vi "VMUIAsync_Viewer.vi"(6 "SetList VariableManager ref":refnum<vi>, 10 "SubPanelRef":refnum<vi>, 11 "VariableManagerRef in":refnum<vi>) -> ()   [LabVIEW 2013]
doc: "Asynchronously call VMUI.vi with the given input. The caller process will not be blocked."
uses:
  VariableManager/VariableManager.lvclass
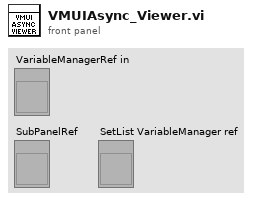
[diagram p1: front panel]
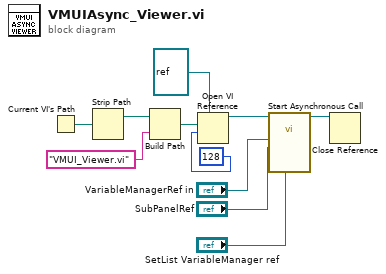
[diagram p0: block diagram]
diagram:
  n1 = Current VI's Path() -> (path=w9:path)
  n2 = Strip Path(path=w9) -> (stripped path=w10:path)  [unwired: 1 out]
  n3 = Build Path(base path=w10, name or relative path="VMUI_Viewer.vi") -> (appended path=w8:path)
  n4 = Open VI Reference(type specifier VI Refnum (for type only)=refnum<vi> refnum, vi path=w8, options=128) -> (vi reference=w4:refnum<vi>)  [unwired: 3 in, 1 out]
  n5 = call-by-ref "Start Asynchronous Call"(reference=w4, "SetList VariableManager Ref in"="SetList VariableManager ref", "SubPanelRef"="SubPanelRef", "VariableManagerRef in"="VariableManagerRef in") -> (reference out=w1:refnum<vi>)  [unwired: 9 in, 2 out]
  n6 = Close Reference(reference=w1) -> ()  [unwired: 1 in, 1 out]
